vi "RespaceForSP.vi"(11 "Code":string) -> (3 "Cleaned for SPIKE":string)   [LabVIEW 2020]
panel:
  out "spreadsheet string":string
  out "Array":i32[](array[numeric])
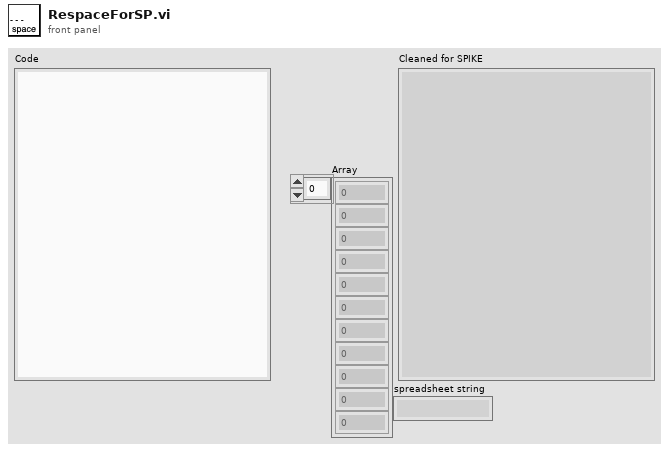
[diagram p1: front panel]
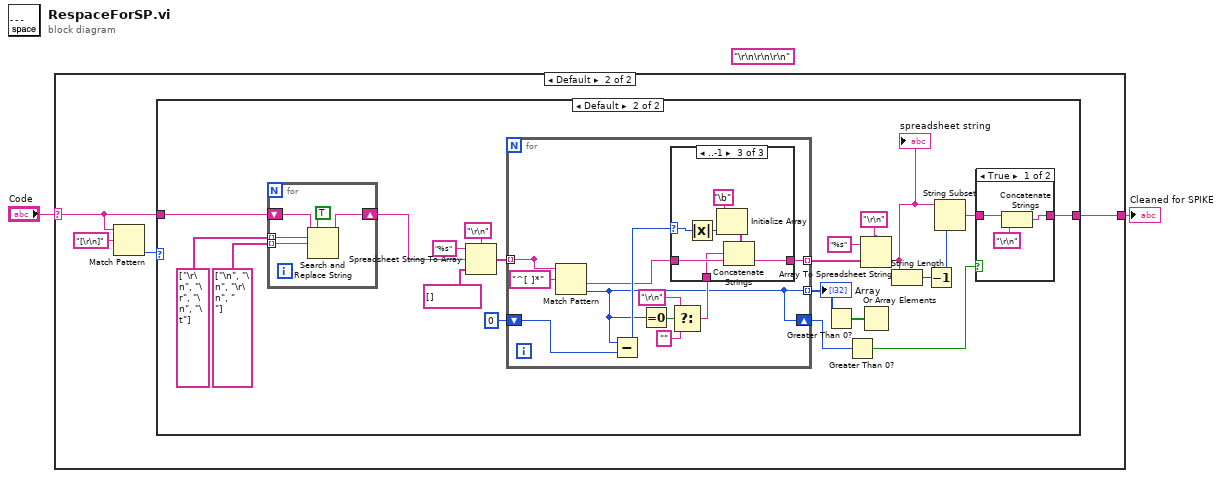
[diagram p0: block diagram]
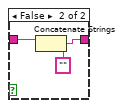
[diagram p4: hidden frame]
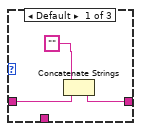
[diagram p5: hidden frame]
diagram:
  (unwired) "\r\n\r\n\r\n" ("replace string (\"\")")
  n1 = case shown="Default" "Code" {
    selector: "Code" -> [w3 w6]
    tunnel: [w3 w4] -> w2
    frame "" {
    }
    frame Default {
      n2 = Match Pattern(string=w6, regular expression="[\r\n]") -> (offset past match=w5:i32)  [unwired: 1 in, 3 out]
      n3 = case shown="Default" w5 {
        tunnel: w6 -> [w8 w29]
        tunnel: [w8 w18] -> w4
        frame -1 {
        }
        frame Default {
          n4 = for {
            tunnel: string[] ["\r\n", "\r", "\n", "\t"] -> [w60] mode=indexing
            tunnel: string[] ["\n", "\n", "\r\n", "    "] -> [w59] mode=indexing
            shift-right: [w58] -> w9
            shift-left: w29 -> [w62]
            n5 = Search and Replace String(replace all?=TRUE ("replace all? (F)"), input string=w62, search string=w60, replace string=w59) -> (result string=w58:string)  [unwired: 4 in, 3 out]
          }
          n6 = Spreadsheet String To Array(delimiter (Tab)="\r\n" ("replace string (\"\")"), format string="%s", spreadsheet string=w9, array type (2D Dbl)=string[] []) -> (array=w23:string[])
          n7 = for {
            tunnel: [w46] -> _ mode=indexing
            tunnel: w23 -> [w46] mode=indexing
            tunnel: [w36] -> w17 mode=indexing
            tunnel: [w42] -> w22 mode=indexing
            shift-right: [w36] -> w11
            shift-left: 0 ("offset past match") -> [w44]
            n8 = Match Pattern(string=w46, regular expression="^[ ]*") -> (after substring=w41:string, offset past match=w36:i32)  [unwired: 1 in, 2 out]
            n9 = Subtract(x=w36, y=w44) -> (x-y=w43:i32)
            n10 = Equal To 0?(x=w36) -> (x = 0?=w40:bool)
            n11 = Select(t="\r\n" ("replace string (\"\")"), s=w40, f="" ("replace string (\"\")")) -> (s? t:f=w37:string)
            n12 = case shown="..-1" w43 {
              selector: w43 -> [_ _ w55]
              tunnel: [w48 w50 w57] -> w42
              tunnel: w41 -> [w49 w50 w56]
              tunnel: w37 -> [_ _ w51]
              frame Default {
                n13 = Concatenate Strings("" ("replace string (\"\")"), w49) -> (w48:string)
              }
              frame 0 {
              }
              frame ..-1 {
                n14 = Absolute Value(x=w55) -> (abs(x)=w53:i32)
                n15 = Initialize Array("\b" ("replace string (\"\")"), w53) -> (w52:string[])
                n16 = Concatenate Strings(w52, w51, w56) -> (w57:string)
              }
            }
          }
          "Array" <- w17
          n17 = Greater Than 0?(x=w17) -> (x > 0?=w16:bool[])
          n18 = Greater Than 0?(x=w11) -> (x > 0?=w10:bool)
          n19 = Array To Spreadsheet String(delimiter (Tab)="\r\n" ("replace string (\"\")"), array=w22, 3:"%s" ("format string")) -> (spreadsheet string=w14:string)
          "spreadsheet string" <- w14
          n20 = Or Array Elements(Boolean array=w16) -> ()  [unwired: 1 out]
          n21 = String Length(string=w14) -> (length=w15:i32)
          n22 = Decrement(x=w15) -> (x-1=w12:i32)
          n23 = String Subset(string=w14, length (rest)=w12) -> (substring=w13:string)  [unwired: 1 in]
          n24 = case shown="True" w10 {
            tunnel: w13 -> [w31 w34]
            tunnel: [w30 w33] -> w18
            frame True {
              n25 = Concatenate Strings(w31, "\r\n" ("replace string (\"\")")) -> (w30:string)
            }
            frame False {
              n26 = Concatenate Strings(w34, "" ("replace string (\"\")")) -> (w33:string)
            }
          }
        }
      }
    }
  }
  "Cleaned for SPIKE" <- w2
